vi "Get Terminal Name with Device Prefix.vi"(8 "error in (no error)":errorcluster, 10 "Local Terminal Name":string, 11 "task/channels in":refnum<k21>) -> (0 "error out":errorcluster, 2 "Terminal Name with Device Prefix":tag, 3 "task out":refnum<k21>)   [LabVIEW 2023]
doc: "This example takes in a DAQmx Task and a terminal and converts this to a terminal which includes the device prefix specified in the DAQmx Physical Channel Control.\n\nFor example: \nDAQmx Task/channels in=Dev1/ai1:2\nTerminal=ai/StartTrigger\nDevice+Terminal=/Dev1/ai/StartTrigger"
uses:
  <resource>/objmgr/daqmx.rc
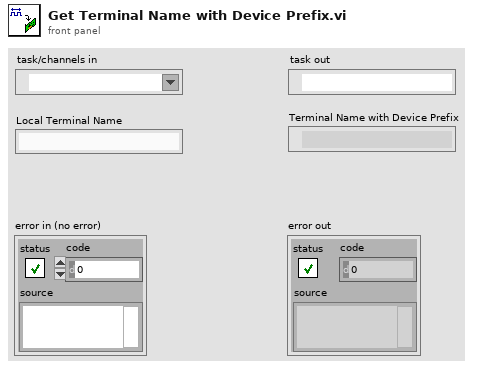
[diagram p1: front panel]
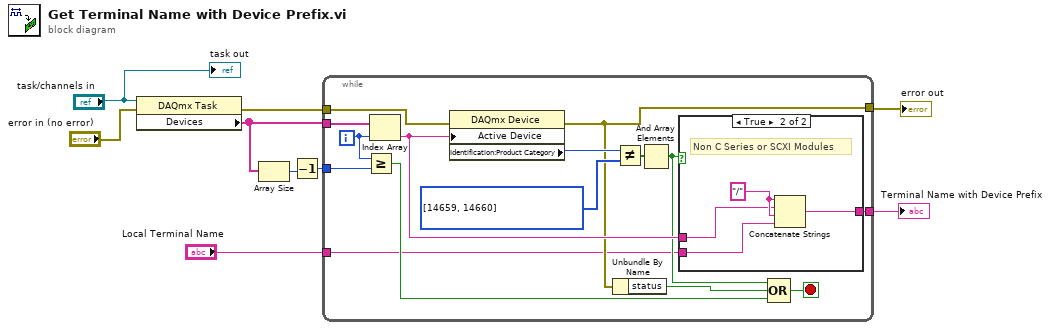
[diagram p0: block diagram]
diagram:
  n1 = property class="DAQmx Task"(reference="task/channels in", error in="error in (no error)") -> (error out=w7:errorcluster, "Devices"=w5:tag[])  [unwired: 1 out]
  n2 = Array Size(array=w5) -> (size(s)=w4:i32)
  n3 = Decrement(x=w4) -> (x-1=w3:i32)
  n4 = while {
    tunnel: w5 -> [w24]
    tunnel: w7 -> [w19]
    tunnel: [w18] -> w6
    tunnel: w3 -> [w16]
    tunnel: "Local Terminal Name" -> [w11]
    tunnel: [w10] -> w1
    i -> [w17]
    stop <- w12 stop-if-true
    w22 = i32[] [14659, 14660] items=["M Series DAQ"=14643, "E Series DAQ"=14642, "S Series DAQ"=14644, "B Series DAQ"=14662, "SC Series DAQ"=14645, "USB DAQ"=14646, "AO Series"=14647, "Digital I/O"=14648, "TIO Series"=14661, "Dynamic Signal Acquisition"=14649, "Switches"=14650, "C Series Chassis"=14658, "C Series Module"=14659, "SCXI Module"=14660, "Unknown"=12588]
    n5 = Greater Or Equal?(x=w17, y=w16) -> (x >= y?=w13:bool)
    n6 = Index Array(array=w24, index=w17) -> (element=w20:tag)
    n7 = property class="DAQmx Device"(error in=w19, "Active Device"=w20) -> (error out=w18:errorcluster, "Identification:Product Category"=w23:i32)  [unwired: 1 in, 1 out]
    n8 = Unbundle By Name(w18) -> ("status"=w14:bool)
    n9 = Not Equal?(x=w23, y=w22) -> (x != y?=w21:bool[])
    n10 = And Array Elements(Boolean array=w21) -> (logical AND=w15:bool)
    n11 = case shown="True" w15 {
      tunnel: w20 -> [_ w25]
      tunnel: w11 -> [_ w27]
      tunnel: [_ w26] -> w10
      frame False {
        # "Module Case do nothing"
      }
      frame True {
        w28 = "/" ("string")
        # "Non C Series or SCXI Modules"
        n12 = Concatenate Strings(w28, w25, w28, w27) -> (w26:string)
      }
    }
    n13 = Compound Arithmetic op=OR(w15, w14, w13) -> (w12:bool)
  }
  "error out" <- w6
  "Terminal Name with Device Prefix" <- w1
  "task out" <- "task/channels in"
